vi "InitSlowCtrlH5.vi"() -> ()   [LabVIEW 2012]
uses:
  <vilib>/addons/h5labview2/file/H5Fmode.ctl
  <vilib>/addons/h5labview2/base/lib_path.vi
  <vilib>/addons/h5labview2/base/H5Equery.vi
  <vilib>/addons/h5labview2/dataset/H5Dwrite.llb/H5Dwrite.xnode
  <vilib>/addons/h5labview2/file/H5F.lvlib
panel:
  in  "Headers":string[](array[string])=["Date\nDate", "Time", "Termination", "RTD0", "RTD1", "RTD2", "RTD3", "RTD4"]
  in  "File Path":path=path "C:/Users/lab-341/Desktop"
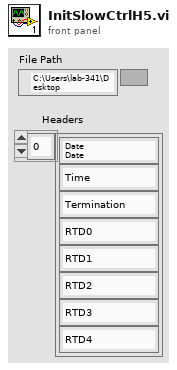
[diagram p1: front panel]
types:
  T1 = typedef "H5F.lvlib/H5Fmode.ctl" = enum16{"read-only", "read-write", "overwrite", "create new", "open or create"}
  T2 = typedef "hid_t.ctl" = i64
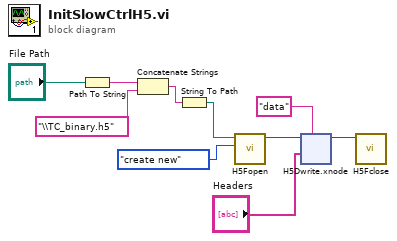
[diagram p0: block diagram]
diagram:
  n1 = Path To String(path="File Path") -> (string=w7:string)
  n2 = Concatenate Strings(w7, "\\TC_binary.h5") -> (w9:string)
  n3 = String To Path(string=w9) -> (path=w6:path)
  n4 = call <vilib>:"H5Fopen.vi"("mode (read-only)"=H5Fmode."create new", "path"=w6) -> ("ref out"=w4:T2)  [unwired: 8 in, 1 out]
  n5 = xnode "H5Dwrite.xnode"("dataset name"="data", "data"="Headers", "ref in"=w4) -> ("ref out"=w3:i64)  [unwired: 4 in, 2 out]
  n6 = call <vilib>:"H5Fclose.vi"("ref"=w3) -> ()  [unwired: 10 in, 1 out]
